vi "MEMR-Create Stimuli.vi"(0 "AO":T2 {"noiseChan"."Filter"."Stages"."IIR Filter"."Forward Coefficients" format="%.4f"; "noiseChan"."Filter"."Stages"."IIR Filter"."Reverse Coefficients" format="%.4f"}, 11 "error in (no error)":errorcluster, 12 "Step In":T1) -> (13 "finished":bool, 14 "Step Out":T1, 15 "error out":errorcluster)   [LabVIEW 2020]
uses:
  Typedefs/MEMR-AO Data.ctl
  Signal Synthesis VIs/3rd Generation/XControls/Stimulus Channel (G3)/Full Stimulus Channel Data.ctl
  Signal Synthesis VIs/3rd Generation/XControls/Waveform XControls/Waveform (G3)/Waveform Data.ctl
  Signal Synthesis VIs/3rd Generation/Waveform VIs/Waveform Enum (V3).ctl
  Signal Synthesis VIs/3rd Generation/XControls/Waveform XControls/Tone (G3)/Tone.Properties.ctl
  Signal Synthesis VIs/Waveform VIs/Pulse Train VIs/Pulse Train Params.ctl
  Signal Synthesis VIs/Waveform VIs/Pulse Train VIs/Pulse Polarity.ctl
  Signal Synthesis VIs/Waveform VIs/Pulse Train VIs/PT-Continuous State.ctl
  Signal Synthesis VIs/3rd Generation/Waveform VIs/Noise VIs/Noise (G3).ctl
  Signal Synthesis VIs/3rd Generation/Waveform VIs/Noise VIs/Noise (G3).Properties.ctl
  Signal Synthesis VIs/3rd Generation/Waveform VIs/Noise VIs/Noise (G3).Data.ctl
  Signal Synthesis VIs/Waveform VIs/File VIs/StimFile-Params.ctl
  Signal Synthesis VIs/Waveform VIs/FM Sweep VIs/FM Sweep Params.ctl
  Signal Synthesis VIs/Waveform VIs/Chirp Train VIs/Chirp Train.ctl
  Signal Synthesis VIs/Waveform VIs/Chirp Train VIs/Chirp Train Params.ctl
  Signal Synthesis VIs/Waveform VIs/Complex Tone VIs/CT-Params.ctl
  Signal Synthesis VIs/Waveform VIs/Complex Tone VIs/CT-Phase Enum.ctl
  Signal Synthesis VIs/Waveform VIs/Complex Tone VIs/CT-Runtime Data.ctl
  Signal Synthesis VIs/3rd Generation/XControls/Waveform XControls/FM Tone/Data.ctl
  Signal Synthesis VIs/3rd Generation/XControls/Waveform XControls/Vowel/Vowel.Properties.ctl
  Signal Synthesis VIs/3rd Generation/Waveform VIs/Ramp VIs/Ramp.Properties.ctl
  Signal Synthesis VIs/3rd Generation/XControls/Filter (G3)/Filter Data.ctl
  Signal Synthesis VIs/3rd Generation/XControls/Filter (G3)/Filter Type.ctl
  Signal Synthesis VIs/Filter VIs/Filter-Bandwidth Units.ctl
  Signal Synthesis VIs/Controls/Burst XCtl/Burst Data.ctl
  Signal Synthesis VIs/3rd Generation/XControls/Level (G3)/Level Data.ctl
  Signal Synthesis VIs/3rd Generation/XControls/Level (G3)/Level Units (G3).ctl
  Signal Synthesis VIs/3rd Generation/XControls/Advanced Options (G3)/Advanced Options (G3).ctl
  Signal Synthesis VIs/Modulation VIs/SAM VIs/SAM Params.ctl
  Signal Synthesis VIs/3rd Generation/Typedefs/Destination.ctl
  Typedefs/MEMR-Sequence Step.ctl
  Signal Synthesis VIs/3rd Generation/XControls/Filter (G3)/Filter (G3).xctl
  Signal Synthesis VIs/3rd Generation/XControls/Level (G3)/Level (G3).xctl
  Signal Synthesis VIs/Controls/Burst XCtl/Burst Control.xctl
  Signal Synthesis VIs/3rd Generation/XControls/Waveform XControls/Tone (G3)/Tone (G3).xctl
  Signal Synthesis VIs/3rd Generation/XControls/Waveform XControls/FM Tone/FM Tone.xctl
  Signal Synthesis VIs/3rd Generation/XControls/Waveform XControls/Vowel/Vowel.xctl
  Signal Synthesis VIs/3rd Generation/XControls/Waveform XControls/Waveform (G3)/Waveform (G3).xctl
  Signal Synthesis VIs/3rd Generation/XControls/Advanced Options (G3)/Advanced Options (G3).xctl
  Signal Synthesis VIs/3rd Generation/XControls/Stimulus Channel (G3)/Stimulus Channel (G3).xctl
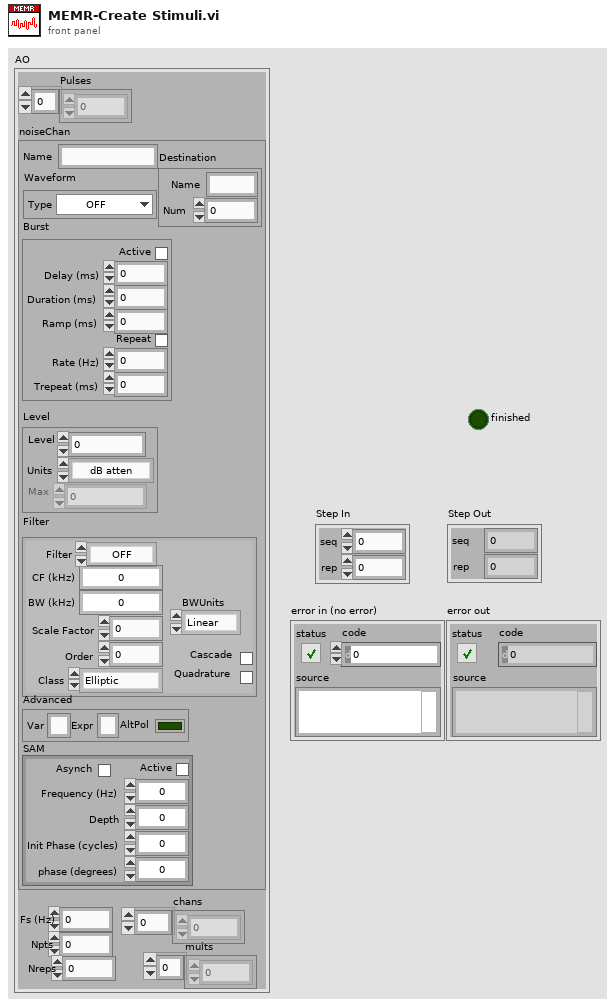
[diagram p1: front panel]
types:
  T1 = typedef "MEMR-Sequence Step.ctl" = cluster{"seq":i32, "rep":i32}
  T2 = typedef "MEMR-AO Data.ctl" = cluster{"Pulses":dbl[], "noiseChan":T3, "Fs (Hz)":dbl, "Npts":i32, "mults":dbl[], "chans":i32[], "Nreps":i32}
  T3 = typedef "Stimulus Channel (G3).xctl/Full Stimulus Channel Data.ctl" = cluster{"Waveform":T4, "Filter":T23, "Burst":T26, "Level":T27, "Name":string, "Advanced":T29, "SAM":T30, "Destination":T31}
  T4 = typedef "Waveform (G3).xctl/Waveform Data.ctl" = cluster{"Type":T5, "Tone":T6, "Pulse Train":T7, "Noise":T10, "File":T13, "FMSweep":T14, "Chirp Train":T15, "Complex Tone":cluster{"Params":T17, "Data":T19}, "FM":T20, "Vowel":T21, "Ramp":T22}
  T5 = typedef "Waveform Enum (V3).ctl" = enum16{"OFF", "Tone", "Noise", "Pulse Train", "File", "FM Sweep", "Chirp Train", "Complex Tone", "FM Tone", "Vowel", "Ramp"}
  T6 = typedef "Tone (G3).xctl/Tone.Properties.ctl" = cluster{"Frequency (kHz)":dbl, "Phase (cycles)":dbl, "Random phase":bool}
  T7 = typedef "Pulse Train Params.ctl" = cluster{"Pulse width (us)":dbl, "Pulse rate (Hz)":dbl, "Gap (ms)":dbl, "Polarity":T8, "PT State":T9, "Asynch":bool}
  T8 = typedef "Pulse Polarity.ctl" = enum16{"POS", "NEG", "POS-NEG", "NEG-POS"}
  T9 = typedef "PT-Continuous State.ctl" = cluster{"Template":dbl[], "Nperiod":i32, "Index":i32, "Pulse Rate (Hz)":dbl, "Phase (cycles)":dbl, "Noff":i32}
  T10 = typedef "Noise (G3).ctl" = cluster{"Properties":T11, "Data":T12}
  T11 = typedef "Noise (G3).Properties.ctl" = cluster{"InvFilt":bool, "Aweight":bool, "Seed":i32, "Tokens":i32, "Brickwall":bool}
  T12 = typedef "Noise (G3).Data.ctl" = cluster{"TokenNum":i32}
  T13 = typedef "StimFile-Params.ctl" = cluster{"Filename":path, "Signal":dbl[], "Channel":i32, "stream":bool, "offset":i32, "nreps":i32, "loops":i32, "Randomize":bool, "order":i32[], "Seed":i32, "Tokens":i32}
  T14 = typedef "FM Sweep Params.ctl" = cluster{"Rate (oct/s)":dbl, "Fmin (Hz)":dbl, "Fmax (Hz)":dbl, "Ramp (ms)":dbl, "Linear":bool}
  T15 = typedef "Chirp Train.ctl" = cluster{"Params":T16, "Data":cluster{"WF":dbl[]}}
  T16 = typedef "Chirp Train Params.ctl" = cluster{"Fmin (kHz)":dbl, "Fmax (kHz)":dbl, "Compensate":bool, "Duration (ms)":dbl}
  T17 = typedef "CT-Params.ctl" = cluster{"F0 (Hz)":dbl, "Band":cluster{"Flow (Hz)":dbl, "Fhigh (Hz)":dbl}, "Phase":T18, "Min F0 (Hz)":dbl, "Max F0 (Hz)":dbl, "ContinRandPhase":bool, "Max peak factor":dbl, "Max mod depth":dbl, "MinHarmNum":i32, "MaxHarmNum":i32, "Level Mode":enum16{"per component", "overall rms"}, "% jitter":dbl}
  T18 = typedef "CT-Phase Enum.ctl" = enum16{"Cosine", "Random", "Alternating"}
  T19 = typedef "CT-Runtime Data.ctl" = cluster{"Ncomp":i32, "MinHarm":i32, "Phase":dbl[], "Amplitude":dbl[], "Npts/frame":i32, "Last F0":dbl, "Fmin":dbl, "Fmax":dbl, "Lslope":dbl, "randphase":bool, "overall rms":bool, "fmult":dbl[], "jittered":bool}
  T20 = typedef "FM Tone.xctl/Data.ctl" = cluster{"Carrier (kHz)":dbl, "ModRate (Hz)":dbl, "Depth (Hz)":dbl, "Phase (cycles)":dbl}
  T21 = typedef "Vowel.xctl/Vowel.Properties.ctl" = cluster{"Freqs":string, "Set level":enum16{"Total", "Per component"}, "Freq":dbl[], "weights":dbl[]}
  T22 = typedef "Ramp.Properties.ctl" = cluster{"Duration (ms)":dbl}
  T23 = typedef "Filter (G3).xctl/Filter Data.ctl" = cluster{"Type":T24, "CF (kHz)":dbl, "BW (kHz)":dbl, "Cascade":bool, "Quadrature":bool, "Scale Factor":dbl, "Stages":cluster{"IIR Filter":cluster{"filter structure":enum32{"IIR 2nd Order", "IIR 4th Order"}, "Reverse Coefficients":dbl[], "Forward Coefficients":dbl[]}, "State":dbl[]}[], "Class":enum16{"Elliptic", "Butterworth"}, "Order":i32, "BWUnits":T25}
  T24 = typedef "Filter (G3).xctl/Filter Type.ctl" = enum16{"OFF", "Lowpass", "Highpass", "Bandpass", "Bandstop"}
  T25 = typedef "Filter-Bandwidth Units.ctl" = enum16{"Linear", "Octaves", "Min-Max"}
  T26 = typedef "Burst Control.xctl/Burst Data.ctl" = cluster{"Active":bool, "Delay (ms)":dbl, "Duration (ms)":dbl, "Ramp (ms)":dbl, "Rate (Hz)":dbl, "Trepeat (ms)":dbl, "Repeat":bool}
  T27 = typedef "Level (G3).xctl/Level Data.ctl" = cluster{"Level":dbl, "Units":T28, "Max":dbl, "Data":cluster{"Multiplier":dbl, "Cal File":path, "Cal":cluster{"Freq (Hz)":dbl[], "Mag (dB SPL)":dbl[], "Phase (deg)":dbl[]}, "audiogram":path}}
  T28 = typedef "Level (G3).xctl/Level Units (G3).ctl" = enum16{"dB atten", "dB SPL", "dB re 1 Vrms", "dB V/Hz½", "mW", "dB HL", "Volts", "dB mW"}
  T29 = typedef "Advanced Options (G3).xctl/Advanced Options (G3).ctl" = cluster{"AltPol":bool, "Var":string, "Expr":string}
  T30 = typedef "SAM Params.ctl" = cluster{"Active":bool, "Frequency (Hz)":dbl, "Depth":dbl, "Init Phase (cycles)":dbl, "phase (degrees)":dbl, "Asynch":bool}
  T31 = typedef "Destination.ctl" = cluster{"Name":string, "Num":i32}
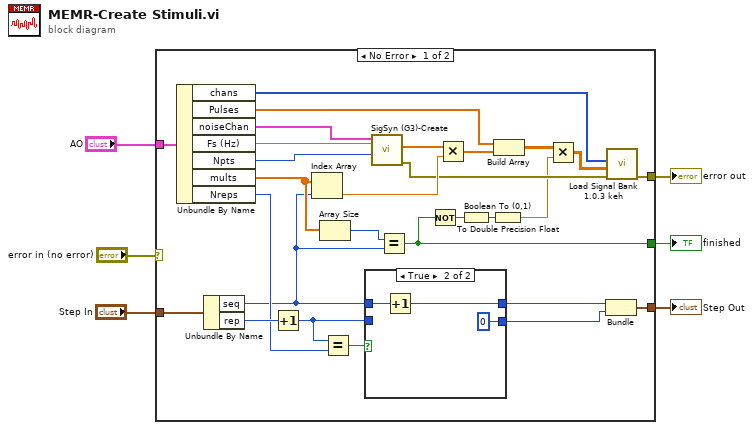
[diagram p0: block diagram]
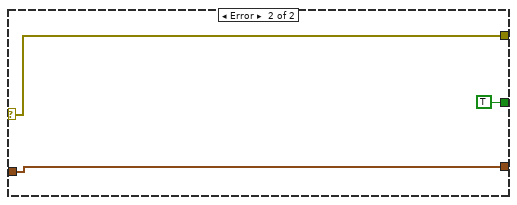
[diagram p3: hidden frame]
diagram:
  n1 = case shown="No Error" "error in (no error)" {
    selector: "error in (no error)" -> [_ w42]
    tunnel: "AO" -> [w34 _]
    tunnel: [w23 w42] -> w5
    tunnel: "Step In" -> [w22 w40]
    tunnel: [w16 w40] -> w2
    tunnel: [w9 TRUE] -> w1
    frame No Error {
      n2 = Unbundle By Name(w34) -> ("chans"=w24:i32[], "Pulses"=w28:dbl[], "noiseChan"=w33:T3, "Fs (Hz)"=w32:dbl, "Npts"=w31:i32, "mults"=w15:dbl[], "Nreps"=w20:i32)
      n3 = Unbundle By Name(w22) -> ("seq"=w12:i32, "rep"=w21:i32)
      n4 = Increment(x=w21) -> (x+1=w18:i32)
      n5 = Index Array(array=w15, index=w12) -> (element=w29:dbl)
      n6 = Array Size(array=w15) -> (size(s)=w13:i32)
      n7 = Equal?(x=w18, y=w20) -> (x = y?=w19:bool)
      n8 = case shown="True" w19 {
        tunnel: w12 -> [w36 w39]
        tunnel: w18 -> [w35 _]
        tunnel: [w36 w38] -> w14
        tunnel: [w35 0] -> w17
        frame False {
        }
        frame True {
          n9 = Increment(x=w39) -> (x+1=w38:i32)
        }
      }
      n10 = call "SigSyn (G3)-Create.vi"("Npts"=w31, "Sampling Rate (Hz)"=w32, "Stimulus Channel"=w33) -> ("error out"=w26:errorcluster, "Waveform"=w30:dbl[])  [unwired: 5 in, 2 out]
      n11 = Equal?(x=w13, y=w12) -> (x = y?=w9:bool)
      n12 = Not(x=w9) -> (.not. x?=w10:bool)
      n13 = Multiply(x=w30, y=w29) -> (x*y=w27:dbl[])
      n14 = Boolean To (0,1)(Boolean=w10) -> (0, 1=w8:i16)
      n15 = To Double Precision Float(number=w8) -> (double precision float=w7:dbl)
      n16 = Build Array(w28, w27) -> (w25:dbl[][])
      n17 = Multiply(x=w25, y=w7) -> (x*y=w11:dbl[][])
      n18 = Bundle("seq"=w14, w17) -> (w16:cluster{"seq":i32, i32})  [unwired: 1 in]
      n19 = call "Load Signal Bank 1.0.3 keh.vi"("error in (no error)"=w26, "Input array"=w11, "Active AO Array"=w24) -> ("error out"=w23:errorcluster)  [unwired: 6 in, 2 out]
    }
    frame Error {
    }
  }
  "error out" <- w5
  "Step Out" <- w2
  "finished" <- w1
